vi "Variant to JSON.vi"(8 "error in":errorcluster, 11 "variant":variant) -> (0 "error out":errorcluster, 3 "concatenated string":string)   [LabVIEW 2011]
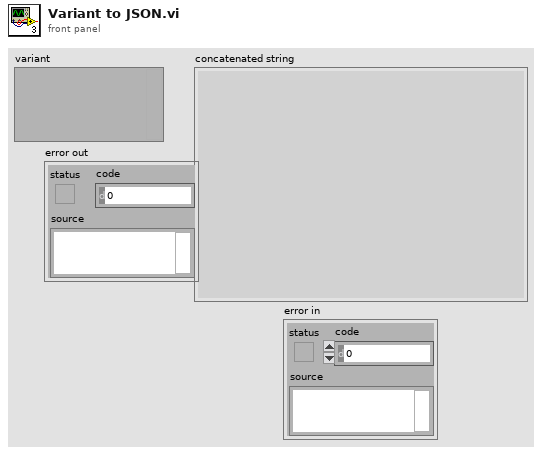
[diagram p1: front panel]
types:
  T1 = typedef "Type Descriptor Enumeration__ogtk.ctl" = enum8{"<Null>", "I8", "I16", "I32", "I64", "U8", "U16", "U32", "U64", "SGL", "DBL", "EXT", "CSG", "CDB", "CXT", "0x0F", "0x10", "0x11", "0x12", "0x13", "0x14", "Enum U8", "Enum U16", "Enum U32", "Enum U64", "SGL PQ", "DBL PQ", "EXT PQ", "CSG PQ", "CDB PQ", "CXT PQ", "0x1F", "0x20", "Boolean", "0x22", "0x23", "0x24", "0x25", "0x26", "0x27", "0x28", "0x29", "0x2A", "0x2B", "0x2C", "0x2D", "0x2E", "0x2F", "String", "0x31", "Path", "Pict", "0x34", "0x35", "0x36", "DAQ", "0x38", "0x39", "0x3A", "0x3B", "0x3C", "0x3D", "0x3E", "0x3F", "Array", "0x41", "0x42", "0x43", "0x44", "0x45", "0x46", "0x47", "0x48", "0x49", "0x4A", "0x4B", "0x4C", "0x4D", "0x4E", "0x4F", "Cluster", "0x51", "0x52", "Variant", "Waveform", "0x55", "0x56", "0x57", "0x58", "0x59", "0x5A", "0x5B", "0x5C", "0x5D", "0x5E", "0x5F", "0x60", "0x61", "0x62", "0x63", "0x64", "0x65", "0x66", "0x67", "0x68", "0x69", "0x6A", "0x6B", "0x6C", "0x6D", "0x6E", "0x6F", "Refnum"}
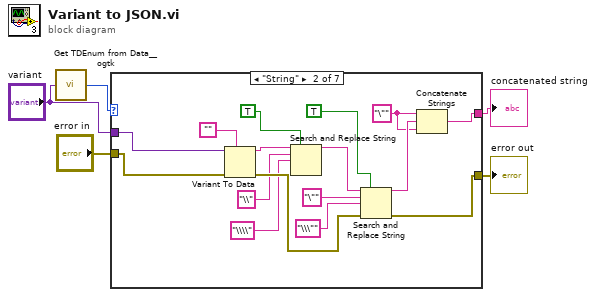
[diagram p0: block diagram]
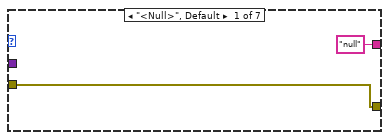
[diagram p2: hidden frame]
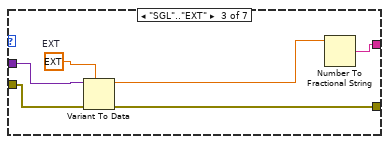
[diagram p3: hidden frame]
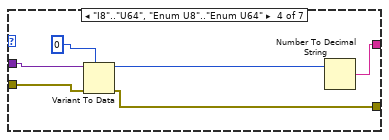
[diagram p4: hidden frame]
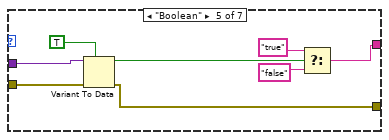
[diagram p5: hidden frame]
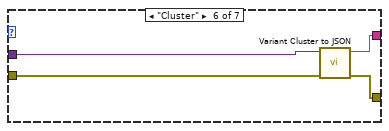
[diagram p6: hidden frame]
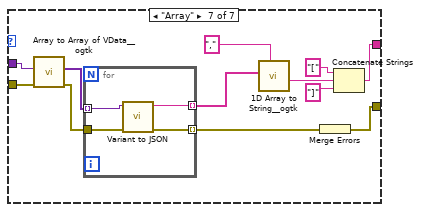
[diagram p7: hidden frame]
diagram:
  n1 = call <userlib>:"Get TDEnum from Data__ogtk.vi"("Data"="variant") -> ("Type Descriptor Enumeration"=w3:T1)  [unwired: 4 in]
  n2 = case shown="\"String\"" w3 {
    tunnel: ["null" ("string") w8 w24 w31 w37 w47 w52] -> w5
    tunnel: "variant" -> [_ w11 w27 w30 w39 w46 w59]
    tunnel: "error in" -> [w6 w10 w26 w33 w38 w45 w50]
    tunnel: [w6 w9 w25 w32 w36 w44 w48] -> w2
    frame "<Null>", Default {
    }
    frame "String" {
      w22 = "\"" ("string")
      n3 = Variant To Data(error in=w10, type="", Variant=w11) -> (data=w16:string, error out=w17:errorcluster)
      n4 = Search and Replace String(replace all?=TRUE ("replace all? (F)"), input string=w16, search string="\\", replace string="\\\\" ("replace string (\"\")")) -> (result string=w12:string)  [unwired: 4 in, 3 out]
      n5 = Search and Replace String(replace all?=TRUE ("replace all? (F)"), input string=w12, search string="\"", replace string="\\\"" ("replace string (\"\")"), error in=w17) -> (result string=w23:string, error out=w9:errorcluster)  [unwired: 3 in, 2 out]
      n6 = Concatenate Strings(w22, w23, w22) -> (w8:string)
    }
    frame "SGL".."EXT" {
      w28 = ext 0.0  # EXT
      n7 = Variant To Data(error in=w26, type=w28, Variant=w27) -> (data=w29:ext, error out=w25:errorcluster)
      n8 = Number To Fractional String(number=w29) -> (F-format string=w24:string)  [unwired: 3 in]
    }
    frame "I8".."U64", "Enum U8".."Enum U64" {
      n9 = Variant To Data(error in=w33, type=i64 0, Variant=w30) -> (data=w35:i64, error out=w32:errorcluster)
      n10 = Number To Decimal String(number=w35) -> (decimal integer string=w31:string)  [unwired: 1 in]
    }
    frame "Boolean" {
      n11 = Variant To Data(error in=w38, type=TRUE, Variant=w39) -> (data=w42:bool, error out=w36:errorcluster)
      n12 = Select(t="true" ("string"), s=w42, f="false" ("string")) -> (s? t:f=w37:string)
    }
    frame "Cluster" {
      n13 = call "Variant Cluster to JSON.vi"("error in"=w45, "Variant"=w46) -> ("error out"=w44:errorcluster, "String"=w47:string)  [unwired: 8 in]
    }
    frame "Array" {
      n14 = call <userlib>:"Array to Array of VData__ogtk.vi"("error in (no error)"=w50, "MultiD Array"=w59) -> ("error out"=w51:errorcluster, "1D Array of Variants"=w58:variant[])  [unwired: 8 in]
      n15 = for {
        tunnel: w58 -> [w63] mode=indexing
        tunnel: [w62] -> w53 mode=indexing
        tunnel: w51 -> [w61]
        tunnel: [w60] -> w49 mode=indexing
        n16 = call "Variant to JSON.vi"("error in"=w61, "variant"=w63) -> ("error out"=w60:errorcluster, "concatenated string"=w62:string)  [unwired: 8 in]
      }
      n17 = call <userlib>:"1D Array to String__ogtk.vi"("delimiter (Tab)"=",", "Array of Strings"=w53) -> ("delimited string"=w57:string)  [unwired: 9 in]
      n18 = Merge Errors(w49) -> (w48:errorcluster)
      n19 = Concatenate Strings("[" ("string"), w57, "]" ("string")) -> (w52:string)
    }
  }
  "concatenated string" <- w5
  "error out" <- w2
